vi "LOAD CELL FGV MAIN.vi"(7 "Enum":T2(ring), 8 "error in (no error)":errorcluster, 11 "main ref":T1) -> (0 "error IO":errorcluster)   [LabVIEW 2025]
uses:
  controls/LAB-IQ UI Data.ctl
  lib/hps_ft.dll
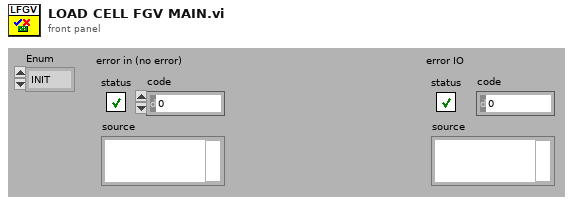
[diagram p1: front panel]
types:
  T1 = typedef "LAB-IQ UI Data.ctl" = cluster{"Main Home Screen":cluster{"GUI":refnum<vi>, "Platform Settings":refnum<vi>, "Configure":refnum<vi>, "Home":refnum<vi>, "EXIT":refnum<vi>, "service 2":refnum<vi>, "MainPage":refnum<vi>, "Analysis":refnum<vi>}, "Platform Settings":cluster{"mm/s  Surge":refnum<vi>, "Update Surge Speed":refnum<vi>, "Drive Error":refnum<vi>, "Disable Axis Jog Soft Limits":refnum<vi>, "mm/s  Sway":refnum<vi>, "Sway and Surge COM Status":refnum<vi>, "Heave COM Status":refnum<vi>, "Enable Platform":refnum<vi>, "Surge Forward Main":refnum<vi>, "Sway Right Main":refnum<vi>, "Sway Left Main":refnum<vi>, "Heave Down Main":refnum<vi>, "Heave Up main":refnum<vi>, "Update Sway Speed":refnum<vi>, "Update Heave Speed":refnum<vi>, "mm/s Heave":refnum<vi>, "mm/sec":refnum<vi>, "mm":refnum<vi>, "Surge Backward Main":refnum<vi>}, "Analysis Screen":cluster{"Analysis Home":refnum<vi>, "Surface Analysis":refnum<vi>, "Imaging":refnum<vi>, "Image Analysis":refnum<vi>, "Post Analysis":refnum<vi>}, "Config Screen":cluster{"Select Load Head":refnum<vi>, "Notes :":refnum<vi>, "FILE":refnum<vi>, "Sample ID :":refnum<vi>, "Operator ID :":refnum<vi>, "Operator Name :":refnum<vi>, "Auto":refnum<vi>}, "Motion Module":cluster{"zNL":refnum<vi>, "NL disp":refnum<vi>, "Rotary Tab":refnum<vi>, "Motion Direction:  3":refnum<vi>, "E.Velocity 2":refnum<vi>, "e.v/ssr 2":refnum<vi>, "Enter Fixed E.Velocity 2":refnum<vi>, "Enter Final SRR 2":refnum<vi>, "Enter initial SRR 2":refnum<vi>, "Enter Fixed SRR 2":refnum<vi>, "Enter the Final E.Velocity (m/s) 2":refnum<vi>, "Enter initial E.Velocity (m/s) 2":refnum<vi>, "Final Speed (RPM) 3":refnum<vi>, "Initial Speed (RPM) 2":refnum<vi>, "Enter the Final Velocity (m/s) 3":refnum<vi>, "Enter initial Velocity (m/s)  3":refnum<vi>, "Ramp Up 2":refnum<vi>, "TEST SELECTION":refnum<vi>, "SPEED SELECTION : ":refnum<vi>, "Angular Oscillation Set":refnum<vi>, "Traction":refnum<vi>, "Step Speed":refnum<vi>, "StepTable For Load-Speed":refnum<vi>, "StepTable For Speed":refnum<vi>, "Surge Forward MM":refnum<vi>, "Surge Backward MM":refnum<vi>, "M3 Image":refnum<vi>, "String 39":refnum<vi>, "Sway Left MM":refnum<vi>, "Sway Right MM":refnum<vi>, "Disable Axis Jog Soft Limits":refnum<vi>, "mm":refnum<vi>, "Heave Down MM":refnum<vi>, "Heave Up MM":refnum<vi>, "Wear Track Diameter (mm)":refnum<vi>, "Set WTD":refnum<vi>, "HomeScratch":refnum<vi>, "HomeRot":refnum<vi>, "PlaceModule":refnum<vi>, "Enter the Angle (Deg)":refnum<vi>, "Enter the Frequency (Hz)":refnum<vi>, "Motion Mode:":refnum<vi>, "LR Sway":refnum<vi>, "Rot Hor":refnum<vi>, "Scratch":refnum<vi>, "LR Cam":refnum<vi>, "MMBack":refnum<vi>, "MMNext":refnum<vi>, "Rot Ver":refnum<vi>, "Rotary Module Selection":refnum<vi>, "calculate rotary":refnum<vi>, "SPEED SELECTION : rotary":refnum<vi>, "Import 2":refnum<vi>, "Save 2":refnum<vi>, "File Path :  2":refnum<vi>, "String 45":refnum<vi>, "StepTable For Speed 3":refnum<vi>, "Enter the Speed(mm/sec)":refnum<vi>, "Enter the Speed(RPM)":refnum<vi>, "Enter Scratch Speed (mm/s):":refnum<vi>, "SwaySpeed Set":refnum<vi>, "Scartch Offset":refnum<vi>, "Motion type:":refnum<vi>, "HomeScratch 2":refnum<vi>, "Enter Scratch length (mm):":refnum<vi>, "Wear Track Diameter":refnum<vi>, "Rotary Speed Exced":refnum<vi>, "Scratch Mode":refnum<vi>, "No of Scratch":refnum<vi>}, "Environmental control":cluster{"Humidity  Status  3":refnum<vi>, "Low Temp  Status  2":refnum<vi>, "TK4 status 2":refnum<vi>, "Stage Temperature":refnum<vi>, "Sample Temperature":refnum<vi>, "Humidity (Amb)":refnum<vi>, "Clear List":refnum<vi>, "Add to list":refnum<vi>, "Wear":refnum<vi>, "Vibration":refnum<vi>, "Humidity (Chamber)":refnum<vi>, "Temperature (Chamber)":refnum<vi>, "ECR ":refnum<vi>, "Temperature (Amb)":refnum<vi>, "Microphone":refnum<vi>, "Acoustic Emission 3":refnum<vi>, "SNext":refnum<vi>, "APBack":refnum<vi>, "Enter the Temperature (°C):":refnum<vi>, "Enter the Stage \nTemperature (°C):":refnum<vi>, "Enter the Humidity (%Rh):":refnum<vi>, "Low Temp":refnum<vi>, "High Temp":refnum<vi>, "Humidity":refnum<vi>, "Sensors Picked":refnum<vi>}, "About Screen":cluster{"Password":refnum<vi>, "Home Service":refnum<vi>, "Advanced Setting":refnum<vi>, "About Tab":refnum<vi>, "ECR Port:":refnum<vi>, "Ramp Port:":refnum<vi>, "Installation/Replacement completed":refnum<vi>, "Loahead":refnum<vi>, "Heave and Surge COM Port:":refnum<vi>, "Sway COM Port:":refnum<vi>, "Temp Modbus:":refnum<vi>, "Humidity Port:":refnum<vi>, "Edit Gain Constants":refnum<vi>, "Save Gain Constants":refnum<vi>}, "Main Screen":cluster{"Main Screen Tab":refnum<vi>, "Angle and Frequency":refnum<vi>, "Stroke (mm)":refnum<vi>, "Angle (Deg)":refnum<vi>, "Main Speed Tab":refnum<vi>, "MTM MOTOR DISPLAY":refnum<vi>, "Disc Speed (m/sec)":refnum<vi>, "Ball Speed (m/sec)":refnum<vi>, "Disc Speed (RPM)":refnum<vi>, "Ball Speed (RPM)":refnum<vi>, "SPEED TAB":refnum<vi>, "Speed (m/sec)":refnum<vi>, "Set Speed (m/sec)":refnum<vi>, "Speed (RPM)":refnum<vi>, "Set Speed":refnum<vi>, "Time Tab":refnum<vi>, "Time ( HH:MM:SS ) 2":refnum<vi>, "Test Duration":refnum<vi>, "Test Duration 4":refnum<vi>, "TEST CYCLE":refnum<vi>, "TOTAL CYCLES":refnum<vi>, "Set Load (N)":refnum<vi>, "Temp Tabs":refnum<vi>, "Heater":refnum<vi>, "TK4 status":refnum<vi>, "ChamberTemp":refnum<vi>, "SetTmp":refnum<vi>, "Controller  Status":refnum<vi>, "ChamberTemp 2":refnum<vi>, "SetTmp 2":refnum<vi>, "Controller  Status 2":refnum<vi>, "ChamberTemp 3":refnum<vi>, "SetTmp 3":refnum<vi>, "Cooling":refnum<vi>, "Load Communication":refnum<vi>, "Ambient \nTemperature":refnum<vi>, "HumCOMStatus":refnum<vi>, "Ambient\n Humidity":refnum<vi>, "Freq (Hz)":refnum<vi>, "Load En":refnum<vi>, "NLt":refnum<vi>, "zNL 2":refnum<vi>, "Humidity On":refnum<vi>, "humidity disp":refnum<vi>, "Set Humidity":refnum<vi>, "NL disp 2":refnum<vi>, "Humidity On 2":refnum<vi>, "humidity disp 2":refnum<vi>, "Set Humidity 2":refnum<vi>, "NL disp 3":refnum<vi>, "AppLoadSeq scratch":refnum<vi>, "Stop Scratch":refnum<vi>, "ClrLog":refnum<vi>, "Trip Log":refnum<vi>, "STOP":refnum<vi>, "Start Test":refnum<vi>, "Test status":refnum<vi>, "AR Led":refnum<vi>, "Data":refnum<vi>, "Health":refnum<vi>, "Sway COM Status":refnum<vi>, "Heave COM Status":refnum<vi>, "Grp Tab":refnum<vi>, "Sub Graph":refnum<vi>, "SD (mm)":refnum<vi>, "Siliding distance Reset Graph":refnum<vi>, "SDGp":refnum<vi>, "Humidity Reset Graph":refnum<vi>, "HumrGp":refnum<vi>, "Acoustic Emission (mV)":refnum<vi>, "Aqucostic Reset Graph":refnum<vi>, "gACQUOS":refnum<vi>, "ECR RESET":refnum<vi>, "ECR":refnum<vi>, "Temperature Reset":refnum<vi>, "Acoustic Emission (mV) 2":refnum<vi>, "Aqucostic Reset Graph 2":refnum<vi>, "gACQUOS 2":refnum<vi>, "ECR RESET 2":refnum<vi>, "ECR 2":refnum<vi>, "Temperature Reset 2":refnum<vi>, "Temperature (deg c)":refnum<vi>, "Speed Reset Graph":refnum<vi>, "Speed Tab":refnum<vi>, "MTM DISC  SPEED":refnum<vi>, "MTM BALL SPEED":refnum<vi>, "speed mm/sec":refnum<vi>, "Hymidity":refnum<vi>, "Humidity Disable trip":refnum<vi>, "CoF Trip  2":refnum<vi>, "Depth Trip":refnum<vi>, "Weart Deapth":refnum<vi>, "Depth Reset Graph":refnum<vi>, "Weart":refnum<vi>, "Depthz":refnum<vi>, "Depth (µm)":refnum<vi>, "WearGp":refnum<vi>, "NL Trip 2":refnum<vi>, "Load pid":refnum<vi>, "Load Disable Trip":refnum<vi>, "Load Reset Graph":refnum<vi>, "NL Display 4":refnum<vi>, "Main Chart 3":refnum<vi>, "BACK":refnum<vi>, "Depth Trip 2":refnum<vi>, "COF TRIP ":refnum<vi>, "Friction Force (N)":refnum<vi>, "FF Reset Graph":refnum<vi>, "FF Disable Trip":refnum<vi>, "FF TRIP":refnum<vi>, "COF Disable Trip":refnum<vi>, "COF Reset Graph":refnum<vi>, "Start Test Temp":refnum<vi>, "zFF":refnum<vi>, "Friction Force (N) Graph":refnum<vi>, "Coefficient of Friction":refnum<vi>, "Scratch Start Test":refnum<vi>, "FF Tab":refnum<vi>, "Cyclic Friction Force (N)":refnum<vi>, "CZ FF":refnum<vi>, "Cyclic Friction Force (N) Graph":refnum<vi>, "Cyclic Coefficient of Friction":refnum<vi>, "Cyclic FF TRIP":refnum<vi>, "Cyclic FF Disable Trip":refnum<vi>, "cyclic COF Disable Trip":refnum<vi>, "cyclic COF TRIP":refnum<vi>, "cyclic COF Reset Graph":refnum<vi>, "Cyclic FF Reset Graph":refnum<vi>, "Test Trip":refnum<vi>, "Multi Scratch Pass":refnum<vi>}, "Loading":cluster{"Indentation":refnum<vi>, "Reference Sample":refnum<vi>, "Load Cell Communication Slide":refnum<vi>, "com 3":refnum<vi>, "com":refnum<vi>, "DecaForce COM Status":refnum<vi>, "Update":refnum<vi>, "Clear 3":refnum<vi>, "seq":refnum<vi>, "Stribeck table":refnum<vi>, "Stribeck Table  For loading":refnum<vi>, "Loading Mode":refnum<vi>, "Enter the Final Load (N)":refnum<vi>, "Enter the CoF Trip":refnum<vi>, "Enter the Friction Force Trip":refnum<vi>, "Enter the Normal load Trip":refnum<vi>, "Enter the Load  (N)":refnum<vi>, "KiloForce":refnum<vi>, "DecaForce ":refnum<vi>, "MicroForce":refnum<vi>, "LHBack":refnum<vi>, "LHNext":refnum<vi>, "Enter the Loading Rate (N/min)":refnum<vi>, "Message":refnum<vi>, "Warning 2":refnum<vi>, "SSP 0.75":refnum<vi>, "SSP 0.5":refnum<vi>, "SSP 0.3":refnum<vi>, "Warning":refnum<vi>, "gui GIF":refnum<vi>, "Communication is established":refnum<vi>, "AppLoad 4":refnum<vi>, "Multipoint":refnum<vi>, "Load Selection":refnum<vi>}, "PID":cluster{"Ramp MulFac":refnum<vi>, "pulses LoadDiffRamp(2..10)":refnum<vi>, "PulseControlRamp(diff<=3N)":refnum<vi>, "SetLoadDeadband(%) Load(0-10N)":refnum<vi>, "PID gains out delay (microForce)":refnum<vi>, "Ramp":refnum<vi>, "Gain 2":refnum<vi>, "pulses LoadDiff(2..10)":refnum<vi>, "pulses LoadDiff(11..50)":refnum<vi>, "PulseControl(diff<=3N)":refnum<vi>, "SetLoadDeadband(%)  2":refnum<vi>, "Dummy Run":refnum<vi>, "Vertical load (N)":refnum<vi>, "AutoTune":refnum<vi>, "Offset 3 ":refnum<vi>, "apply load":refnum<vi>, "Offset  3":refnum<vi>, "apply load 2":refnum<vi>, "Enter ByPass Load":refnum<vi>, "reinit 3":refnum<vi>, "output range delay":refnum<vi>, "PID gains out delay":refnum<vi>, "Bypass Load":refnum<vi>, "pulsesSent":refnum<vi>, "pulses ":refnum<vi>, "actpid":refnum<vi>, "gFF Rot":refnum<vi>, "pulses LoadDiff(21..1000)":refnum<vi>, "Delay":refnum<vi>, "deadband":refnum<vi>}, "Config Parameters":cluster{"Tab Control 3":refnum<vi>, "Tab Control 19":refnum<vi>, "SAMPLES":refnum<vi>, "Re-initilaize":refnum<vi>, "Filter ON/OFF":refnum<vi>, "TracHomeSurgeOffsetCounts 10MM":refnum<vi>, "TracHomeSwayOffsetCounts 10MM":refnum<vi>, "Acoustic Emission:":refnum<vi>, "Apply Filter (FF)":refnum<vi>, "Filter% 2":refnum<vi>, "Apply Filter (Load)":refnum<vi>, "Filter% ":refnum<vi>, "Sway distance (mm)":refnum<vi>, "Surge distance (mm)":refnum<vi>, "DataSavingLoopDelay(ms)":refnum<vi>, "SAVE 2":refnum<vi>, "Enter Distance":refnum<vi>, "Sway Counts:":refnum<vi>, "Distance (mm): 3":refnum<vi>, "Surge Counts:":refnum<vi>, "Distance (mm): 2":refnum<vi>, "Distance (mm):":refnum<vi>, "Heave Counts:":refnum<vi>, "LRMHomeSurgeOffsetCounts":refnum<vi>, "LRMHomeSwayOffsetCounts":refnum<vi>, "TracHomeSurgeOffsetCounts 20MM":refnum<vi>, "TracHomeSwayOffsetCounts 20MM":refnum<vi>, "RotHomeSwayOffsetCounts":refnum<vi>, "RotHomeSurgeOffsetCounts":refnum<vi>, "Heave distance":refnum<vi>, "Zmm":refnum<vi>, "Heave Pulses/mm":refnum<vi>, "Surge Pulses/mm":refnum<vi>, "Sway Pulses/mm":refnum<vi>, "Heave Pitch":refnum<vi>, "Surge Pitch":refnum<vi>, "Sway Pitch":refnum<vi>, "Heave PPR":refnum<vi>, "Surge PPR":refnum<vi>, "Sway PPR":refnum<vi>, "Tab Control 5":refnum<vi>, "Tab Control 14":refnum<vi>, "Tab Control 26":refnum<vi>, "AE":refnum<vi>, "Heave Loop Delay":refnum<vi>, "Heave PID Speed":refnum<vi>, "Surge Jog Speed":refnum<vi>, "Heave Jog Speed":refnum<vi>, "Sway Loop Delay":refnum<vi>, "Sway PID Speed":refnum<vi>, "Sway Jog Speed":refnum<vi>}, "Loading Com Port":cluster{"ClearAll":refnum<vi>, "Mz(Nm)":refnum<vi>, "My(Nm)":refnum<vi>, "Mx(Nm)":refnum<vi>, "Save Dwell":refnum<vi>, "Mx ":refnum<vi>, "My ":refnum<vi>, "Mz":refnum<vi>, "Fx(N)":refnum<vi>, "Fy(N)":refnum<vi>, "Fz(N)":refnum<vi>, "ZeroAll":refnum<vi>, "Acq Delay (ms)":refnum<vi>, "Burst Delay (ms)":refnum<vi>, "model":refnum<vi>, "SN":refnum<vi>, "FFx(N)":refnum<vi>, "Sensor IP":refnum<vi>, "Port":refnum<vi>, "FFy(N)":refnum<vi>, "Load(N)":refnum<vi>, "delete Handle":refnum<vi>, "Create Handle":refnum<vi>, "ft_data":refnum<vi>, "ft_range":refnum<vi>, "ft_data 2":refnum<vi>, "stop 6":refnum<vi>, "running_flag":refnum<vi>, "ft_udp_handle":refnum<vi>, "get-data-return":refnum<vi>, "get-range-return":refnum<vi>, "zero-return":refnum<vi>, "filter-return":refnum<vi>, "initial-return":refnum<vi>, "deleteHandle-result":refnum<vi>, "Load Cell Temp":refnum<vi>}, "Heave AND Surge":cluster{"SURGE POSE":refnum<vi>, "error out Read":refnum<vi>, "HEAVE POSE":refnum<vi>, "State":refnum<vi>, "Homed":refnum<vi>, "Sequence ID":refnum<vi>, "error out Write":refnum<vi>, "faultCode":refnum<vi>, "Ack ID":refnum<vi>, "SPEED":refnum<vi>, "Distance":refnum<vi>, "Mode Command":refnum<vi>, "Heave and Surge Read":refnum<vi>, "Read Heave Temp":refnum<vi>, "Spare 15":refnum<vi>, "Spare 14":refnum<vi>, "Spare 13":refnum<vi>, "Spare 12":refnum<vi>, "Spare 11":refnum<vi>, "Spare 10":refnum<vi>, "Spare 9":refnum<vi>, "Spare 8":refnum<vi>, "Spare 7":refnum<vi>, "Spare 6":refnum<vi>, "Spare 5":refnum<vi>, "Spare 4":refnum<vi>, "Spare 2":refnum<vi>, "Spare 1":refnum<vi>, "Node Id":refnum<vi>, "Spare 3":refnum<vi>, "SPARE 4":refnum<vi>, "SPARE 3":refnum<vi>, "SPARE 2":refnum<vi>, "SPARE 1":refnum<vi>, "fwMajor":refnum<vi>, "fwMinor":refnum<vi>, "Manual Write":refnum<vi>, "Heave and Surge Write":refnum<vi>}, "New PID LOGIC":cluster{"Fine Tune Zone":refnum<vi>, "PID SDelay":refnum<vi>, "Max_pos_limit":refnum<vi>, "Min_pos_limit":refnum<vi>, "i_limit":refnum<vi>, "pct_scale":refnum<vi>, "Deadband":refnum<vi>, "Kd":refnum<vi>, "Ki":refnum<vi>, "Kp":refnum<vi>, "Current Position":refnum<vi>, "Set Load":refnum<vi>, "Current Load":refnum<vi>, "Pulse delta":refnum<vi>, "Init Step":refnum<vi>, "Max Step Linit":refnum<vi>}, "SWAY ":cluster{"fwMajor":refnum<vi>, "Homed":refnum<vi>, "Rotary POSE":refnum<vi>, "State":refnum<vi>, "SWAY POSE":refnum<vi>, "Ack ID":refnum<vi>, "faultCode":refnum<vi>, "Node Id":refnum<vi>, "fwMinor":refnum<vi>, "Spare 6":refnum<vi>, "Spare 5":refnum<vi>, "Spare 4":refnum<vi>, "Spare 3":refnum<vi>, "Spare 2":refnum<vi>, "Spare 1":refnum<vi>, "Spare 7":refnum<vi>, "SPARE  5":refnum<vi>, "error out Write  SWAY ":refnum<vi>, "error out Read SWAY ":refnum<vi>, "Manual Write SWAY ":refnum<vi>, "SWAY WRITE":refnum<vi>, "SPARE  4":refnum<vi>, "SPARE  3":refnum<vi>, "SPARE 2":refnum<vi>, "SPARE 1":refnum<vi>, "Spare 15":refnum<vi>, "Spare 14":refnum<vi>, "Spare 13":refnum<vi>, "Spare 12":refnum<vi>, "Spare 11":refnum<vi>, "Spare 9":refnum<vi>, "Spare 8":refnum<vi>, "SPEED":refnum<vi>, "Distance":refnum<vi>, "Mode Command":refnum<vi>, "Sequence ID":refnum<vi>, "SWAY READ":refnum<vi>, "Spare 10":refnum<vi>, "Read SWAY Temp":refnum<vi>}, "Analysis Screen":cluster{"Analysis Home":refnum<vi>, "Refresh 2":refnum<vi>, "MEAN 4":refnum<vi>, "SD 4":refnum<vi>, "VARIANCE 4":refnum<vi>, "MEAN  3":refnum<vi>, "SD  3":refnum<vi>, "VARIANCE  3":refnum<vi>, "MEAN 2":refnum<vi>, "SD  2":refnum<vi>, "VARIANCE 2":refnum<vi>, "MEAN":refnum<vi>, "SD":refnum<vi>, "VARIANCE":refnum<vi>, "File 4 Discription":refnum<vi>, "OPEN 4":refnum<vi>, "File Name 4":refnum<vi>, "OPEN 3":refnum<vi>, "File 3 Discription":refnum<vi>, "File Name 3":refnum<vi>, "Y-AXIS":refnum<vi>, "X-AXIS":refnum<vi>, "XY Graph":refnum<vi>, "File Name 2":refnum<vi>, "File Name 1":refnum<vi>, "OPEN 2":refnum<vi>, "OPEN 1":refnum<vi>, "File 1 Discription ":refnum<vi>, "File 2 Discription":refnum<vi>}}
  T2 = enum16{"INIT", "SETLOWPASSFILTER", "SETZERO", "GETSENSORINFO", "GETRANGE", "ZEROALL", "READDATA", "UNINITIAL", "DELETEHANDLE"}
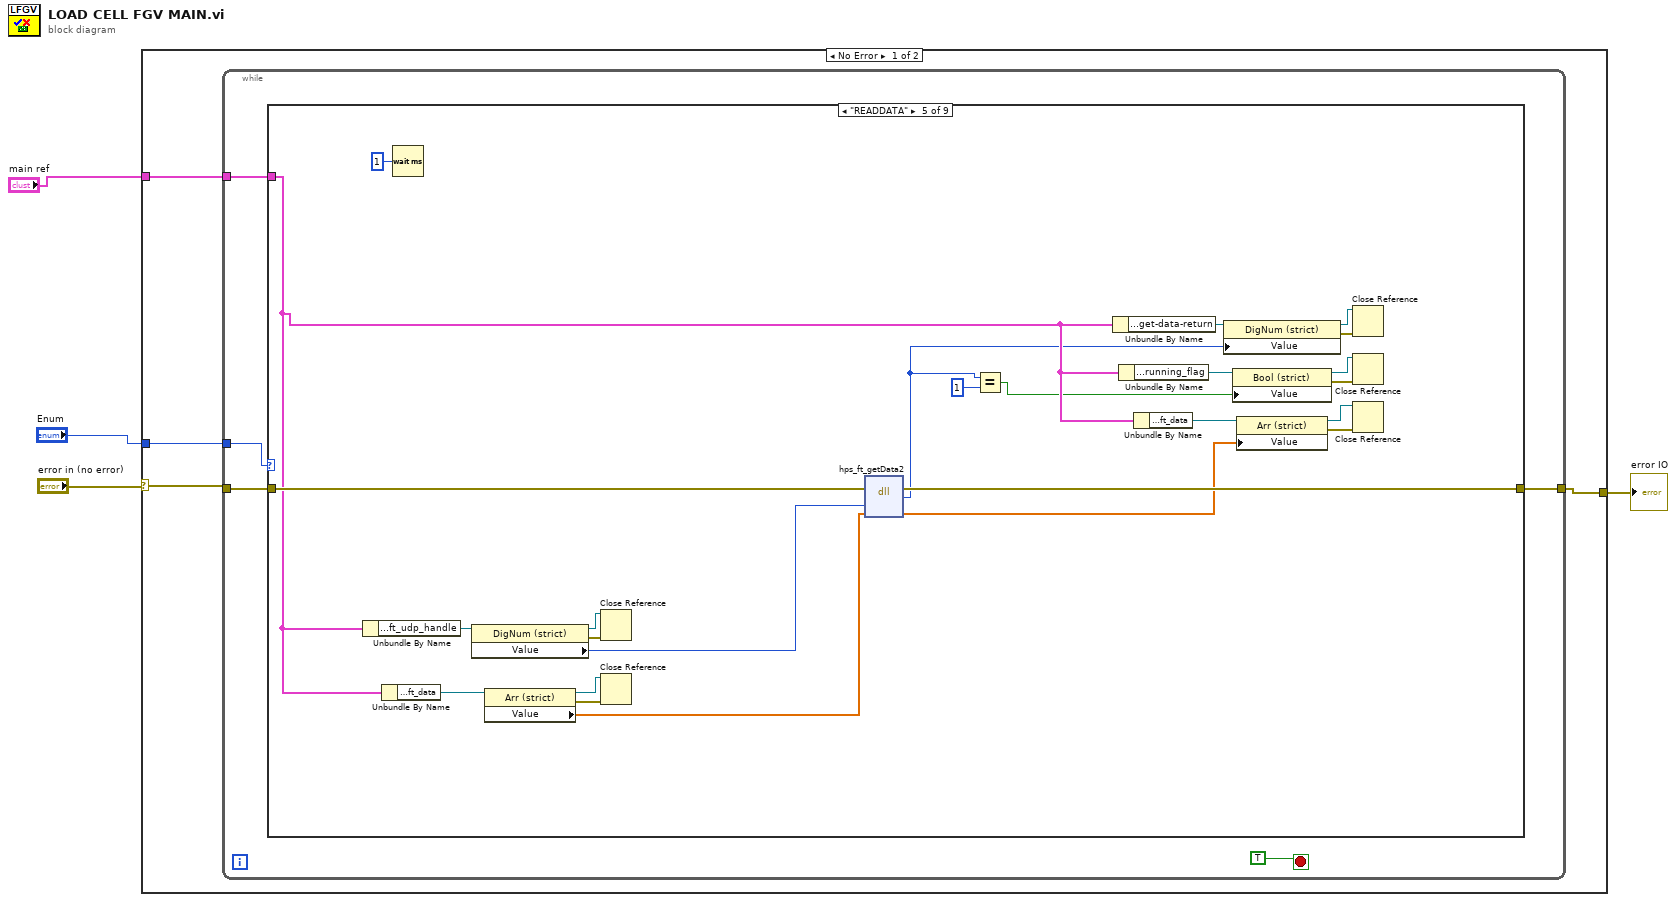
[diagram p0: block diagram]
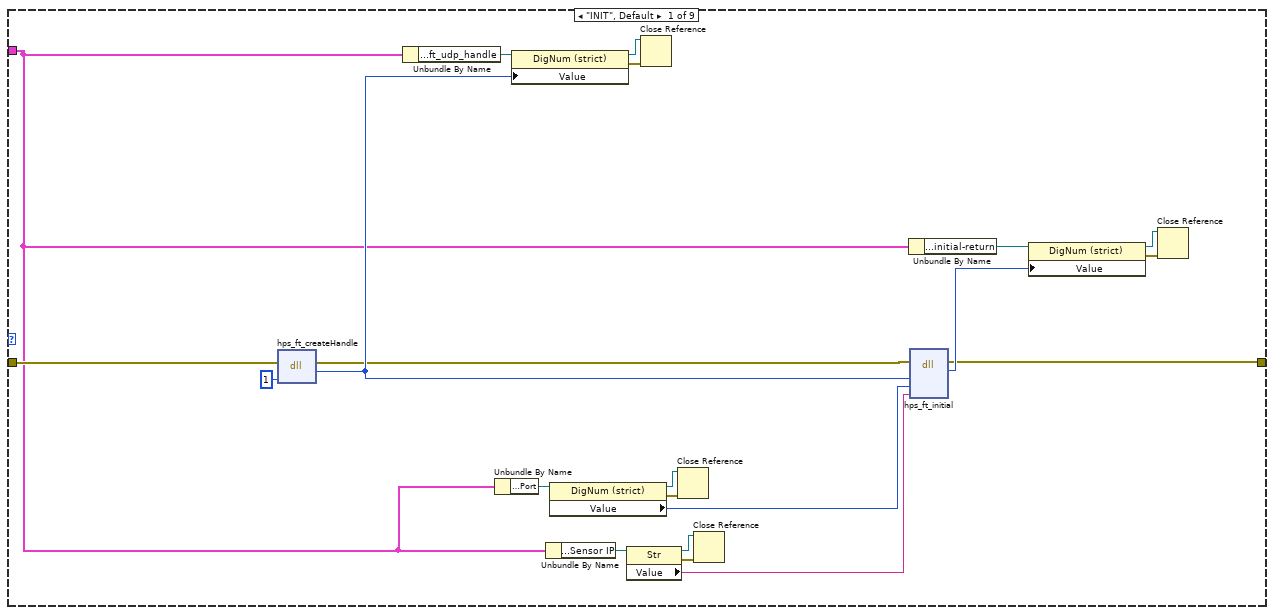
[diagram p2: hidden frame]
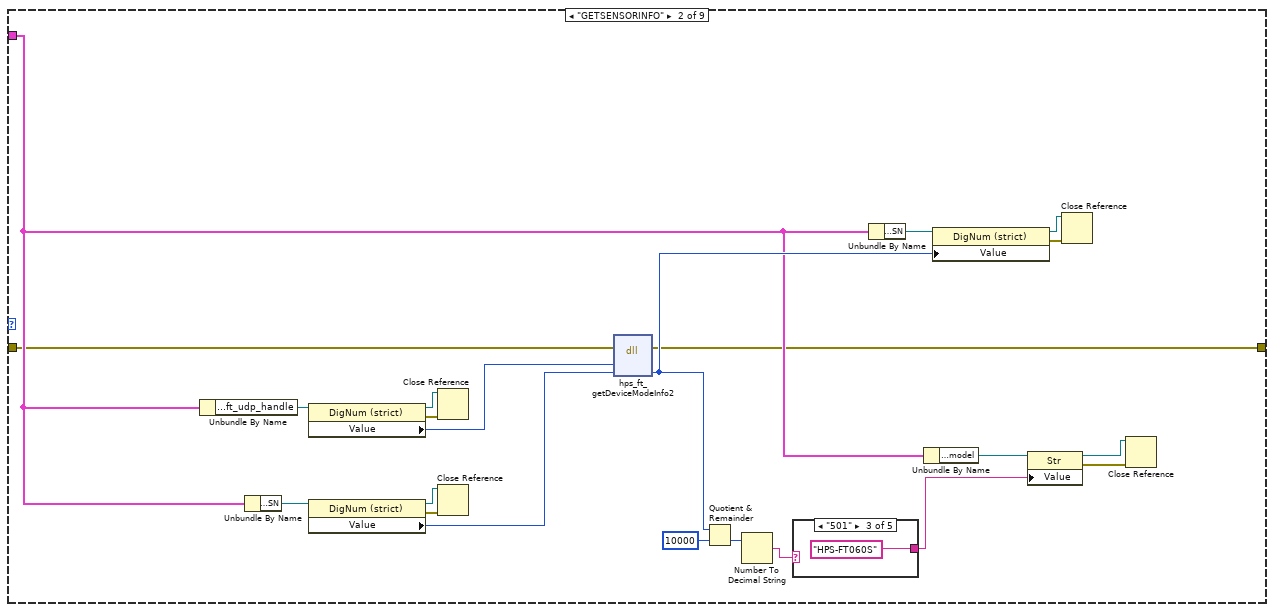
[diagram p3: hidden frame]
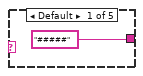
[diagram p4: hidden frame]
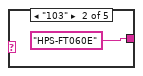
[diagram p5: hidden frame]
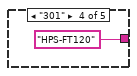
[diagram p6: hidden frame]
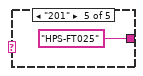
[diagram p7: hidden frame]
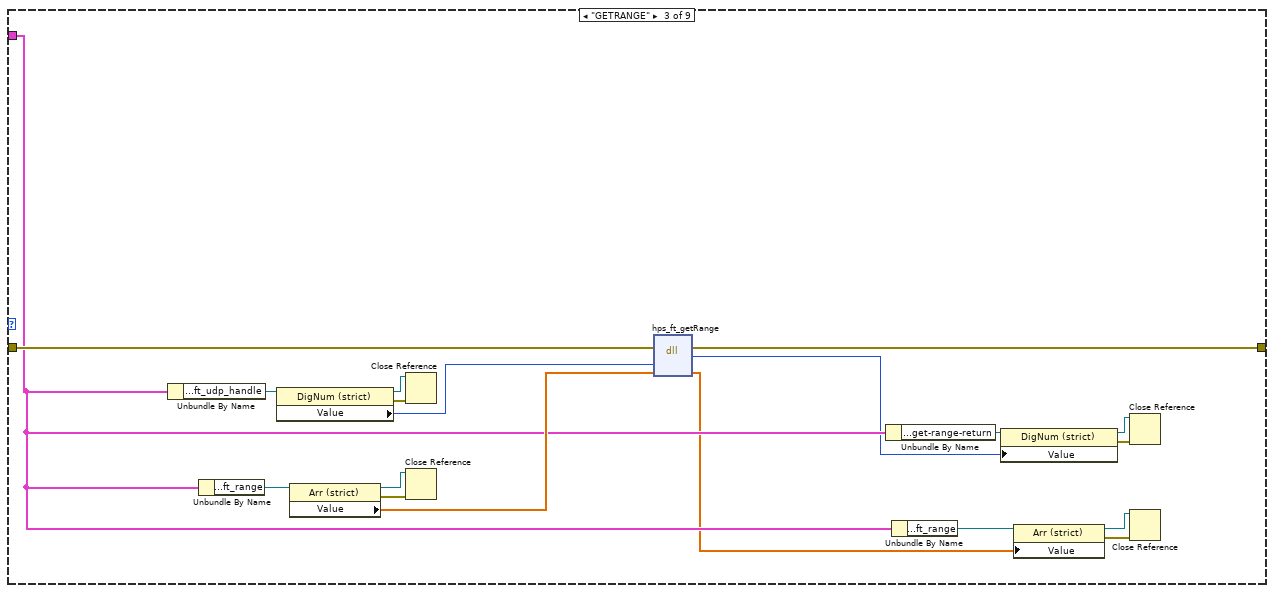
[diagram p8: hidden frame]
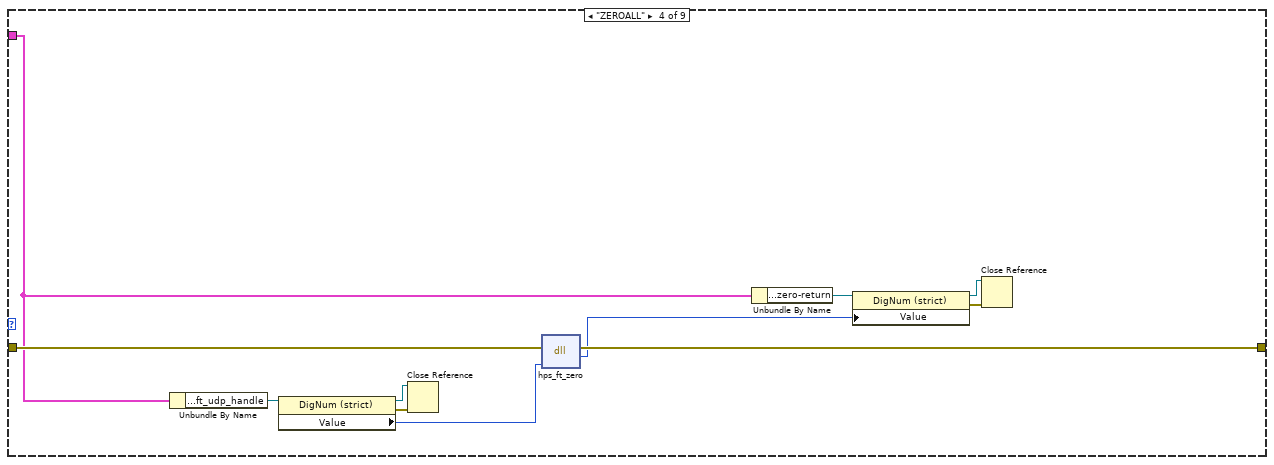
[diagram p9: hidden frame]
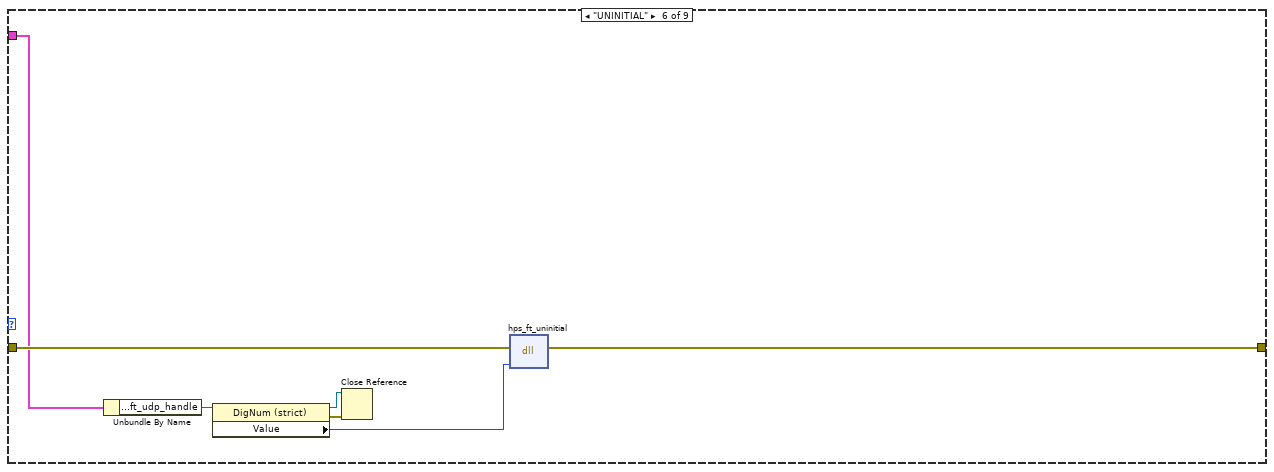
[diagram p10: hidden frame]
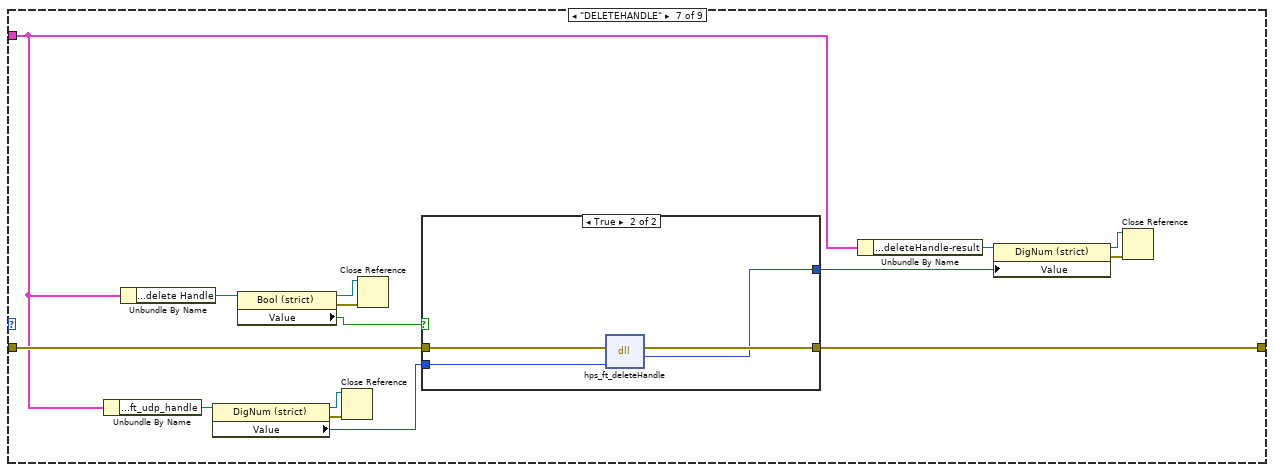
[diagram p11: hidden frame]
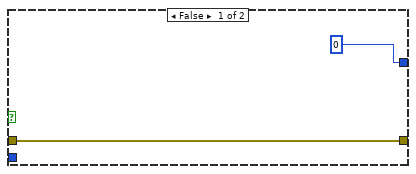
[diagram p12: hidden frame]
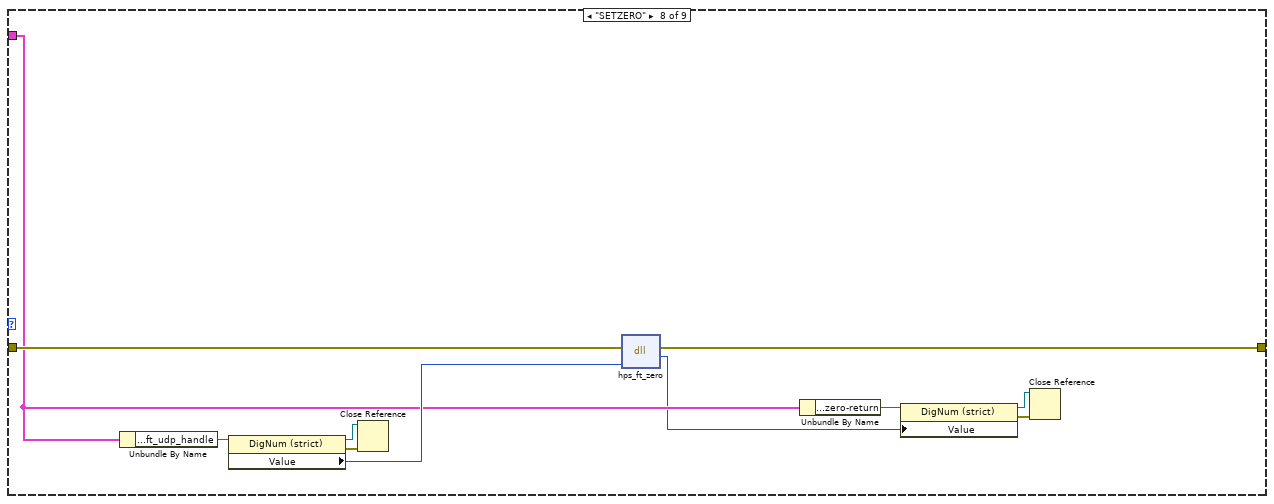
[diagram p13: hidden frame]
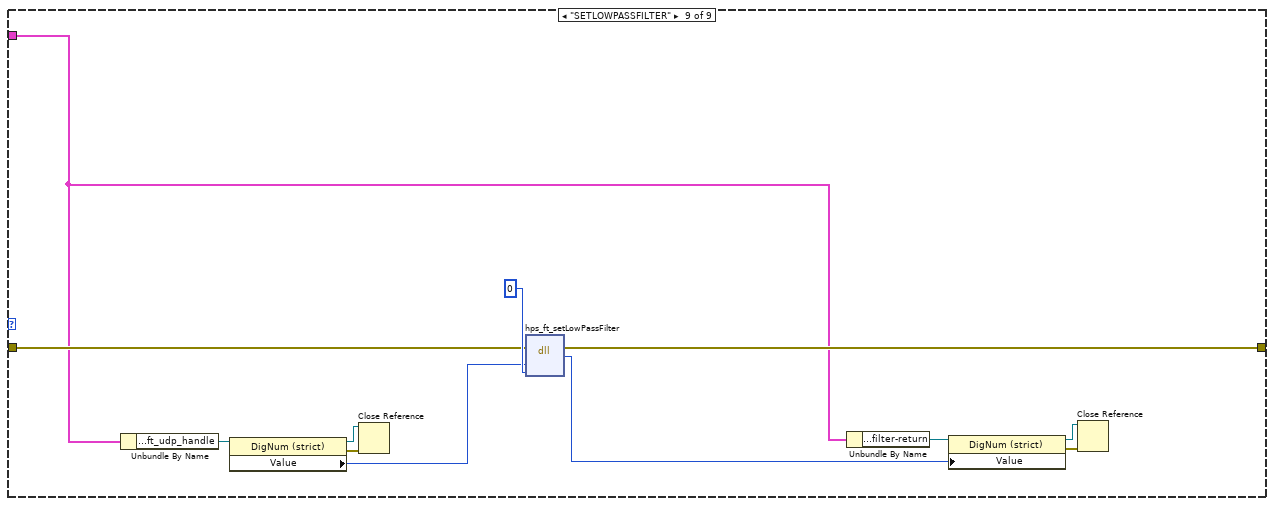
[diagram p14: hidden frame]
diagram:
  n1 = case shown="No Error" "error in (no error)" {
    selector: "error in (no error)" -> [w8 _]
    tunnel: [w7 _] -> w3
    tunnel: "Enum" -> [w6 _]
    tunnel: "main ref" -> [w5 _]
    frame No Error {
      n2 = while {
        tunnel: [w11] -> w7
        tunnel: w8 -> [w12]
        tunnel: w6 -> [w10]
        tunnel: w5 -> [w9]
        stop <- TRUE ("stop") stop-if-true
        n3 = case shown="\"READDATA\"" w10 {
          tunnel: w12 -> [w21 w36 w80 w91 w114 w123 w138 w155 w166]
          tunnel: [w14 w35 w79 w90 w113 w122 w137 w145 w165] -> w11
          tunnel: w9 -> [w16 w38 w64 w82 w96 w117 w125 w147 w157]
          frame "INIT", Default {
            n4 = dll-call lib="D:/LAB-IQ 150/lib/hps_ft.dll" fn="hps_ft_createHandle"(error in=w21, "1(UDP)"=1) -> (error out=w20:errorcluster, "return type"=w30:i32)  [unwired: 3 in, 1 out]
            n5 = Unbundle By Name(w16) -> ("Loading Com Port.ft_udp_handle"=w31:refnum<vi>)
            n6 = Unbundle By Name(w16) -> ("Loading Com Port.Port"=w25:refnum<vi>)
            n7 = property class="DigNum (strict)"(reference=w31, "Value"=w30) -> (reference out=w33:refnum<vi>, error out=w32:errorcluster)  [unwired: 1 in]
            n8 = Unbundle By Name(w16) -> ("Loading Com Port.Sensor IP"=w29:refnum<vi>)
            n9 = property class="DigNum (strict)"(reference=w25) -> (reference out=w24:refnum<vi>, error out=w26:errorcluster, "Value"=w23:i32)  [unwired: 1 in]
            n10 = property class="Str"(reference=w29) -> (reference out=w27:refnum<vi>, error out=w28:errorcluster, "Value"=w22:string)  [unwired: 1 in]
            n11 = Close Reference(reference=w33, error in (no error)=w32) -> ()  [unwired: 1 out]
            n12 = Close Reference(reference=w24, error in (no error)=w26) -> ()  [unwired: 1 out]
            n13 = Close Reference(reference=w27, error in (no error)=w28) -> ()  [unwired: 1 out]
            n14 = Unbundle By Name(w16) -> ("Loading Com Port.initial-return"=w19:refnum<vi>)
            n15 = dll-call lib="D:/LAB-IQ 150/lib/hps_ft.dll" fn="hps_ft_initial"(error in=w20, "handle"=w30, "port"=w23, "IP"=w22) -> (error out=w14:errorcluster, "return type"=w15:i32)  [unwired: 5 in, 1 out]
            n16 = property class="DigNum (strict)"(reference=w19, "Value"=w15) -> (reference out=w17:refnum<vi>, error out=w18:errorcluster)  [unwired: 1 in]
            n17 = Close Reference(reference=w17, error in (no error)=w18) -> ()  [unwired: 1 out]
          }
          frame "GETSENSORINFO" {
            n18 = Unbundle By Name(w38) -> ("Loading Com Port.ft_udp_handle"=w51:refnum<vi>)
            n19 = Unbundle By Name(w38) -> ("Loading Com Port.SN"=w48:refnum<vi>)
            n20 = property class="DigNum (strict)"(reference=w51) -> (reference out=w53:refnum<vi>, error out=w52:errorcluster, "Value"=w47:i32)  [unwired: 1 in]
            n21 = property class="DigNum (strict)"(reference=w48) -> (reference out=w50:refnum<vi>, error out=w49:errorcluster, "Value"=w46:i32)  [unwired: 1 in]
            n22 = Close Reference(reference=w53, error in (no error)=w52) -> ()  [unwired: 1 out]
            n23 = Close Reference(reference=w50, error in (no error)=w49) -> ()  [unwired: 1 out]
            n24 = dll-call lib="D:/LAB-IQ 150/lib/hps_ft.dll" fn="hps_ft_getDeviceModeInfo2"(error in=w36, "handle"=w47, "sensor_info"=w46) -> (error out=w35:errorcluster, "sensor_info"=w42:i32)  [unwired: 4 in, 1 out]
            n25 = Quotient & Remainder(x=w42, y=10000) -> (floor(x/y)=w56:i32)  [unwired: 1 out]
            n26 = Number To Decimal String(number=w56) -> (decimal integer string=w54:string)  [unwired: 1 in]
            n27 = case shown="\"501\"" w54 {
              tunnel: ["#####" "HPS-FT060E" "HPS-FT060S" "HPS-FT120" "HPS-FT025"] -> w37
              frame Default {
              }
              frame "103" {
              }
              frame "501" {
              }
              frame "301" {
              }
              frame "201" {
              }
            }
            n28 = Unbundle By Name(w38) -> ("Loading Com Port.SN"=w45:refnum<vi>)
            n29 = Unbundle By Name(w38) -> ("Loading Com Port.model"=w39:refnum<vi>)
            n30 = property class="DigNum (strict)"(reference=w45, "Value"=w42) -> (reference out=w43:refnum<vi>, error out=w44:errorcluster)  [unwired: 1 in]
            n31 = property class="Str"(reference=w39, "Value"=w37) -> (reference out=w41:refnum<vi>, error out=w40:errorcluster)  [unwired: 1 in]
            n32 = Close Reference(reference=w43, error in (no error)=w44) -> ()  [unwired: 1 out]
            n33 = Close Reference(reference=w41, error in (no error)=w40) -> ()  [unwired: 1 out]
          }
          frame "GETRANGE" {
            n34 = Unbundle By Name(w64) -> ("Loading Com Port.ft_udp_handle"=w76:refnum<vi>)
            n35 = Unbundle By Name(w64) -> ("Loading Com Port.ft_range"=w73:refnum<vi>)
            n36 = property class="DigNum (strict)"(reference=w76) -> (reference out=w78:refnum<vi>, error out=w77:errorcluster, "Value"=w72:i32)  [unwired: 1 in]
            n37 = property class="Arr (strict)"(reference=w73) -> (reference out=w75:refnum<vi>, error out=w74:errorcluster, "Value"=w71:dbl[])  [unwired: 1 in]
            n38 = Close Reference(reference=w78, error in (no error)=w77) -> ()  [unwired: 1 out]
            n39 = Close Reference(reference=w75, error in (no error)=w74) -> ()  [unwired: 1 out]
            n40 = dll-call lib="D:/LAB-IQ 150/lib/hps_ft.dll" fn="hps_ft_getRange"(error in=w80, "handle"=w72, "fi_data"=w71) -> (error out=w79:errorcluster, "return type"=w62:i32, "fi_data"=w63:dbl[])  [unwired: 3 in, 1 out]
            n41 = Unbundle By Name(w64) -> ("Loading Com Port.get-range-return"=w68:refnum<vi>)
            n42 = Unbundle By Name(w64) -> ("Loading Com Port.ft_range"=w65:refnum<vi>)
            n43 = property class="DigNum (strict)"(reference=w68, "Value"=w62) -> (reference out=w70:refnum<vi>, error out=w69:errorcluster)  [unwired: 1 in]
            n44 = property class="Arr (strict)"(reference=w65, "Value"=w63) -> (reference out=w67:refnum<vi>, error out=w66:errorcluster)  [unwired: 1 in]
            n45 = Close Reference(reference=w70, error in (no error)=w69) -> ()  [unwired: 1 out]
            n46 = Close Reference(reference=w67, error in (no error)=w66) -> ()  [unwired: 1 out]
          }
          frame "ZEROALL" {
            n47 = Unbundle By Name(w82) -> ("Loading Com Port.ft_udp_handle"=w87:refnum<vi>)
            n48 = property class="DigNum (strict)"(reference=w87) -> (reference out=w89:refnum<vi>, error out=w88:errorcluster, "Value"=w86:i32)  [unwired: 1 in]
            n49 = Close Reference(reference=w89, error in (no error)=w88) -> ()  [unwired: 1 out]
            n50 = dll-call lib="D:/LAB-IQ 150/lib/hps_ft.dll" fn="hps_ft_zero"(error in=w91, "handle"=w86) -> (error out=w90:errorcluster, "return type"=w81:i32)  [unwired: 3 in, 1 out]
            n51 = Unbundle By Name(w82) -> ("Loading Com Port.zero-return"=w83:refnum<vi>)
            n52 = property class="DigNum (strict)"(reference=w83, "Value"=w81) -> (reference out=w85:refnum<vi>, error out=w84:errorcluster)  [unwired: 1 in]
            n53 = Close Reference(reference=w85, error in (no error)=w84) -> ()  [unwired: 1 out]
          }
          frame "READDATA" {
            n54 = Unbundle By Name(w96) -> ("Loading Com Port.ft_udp_handle"=w110:refnum<vi>)
            n55 = Unbundle By Name(w96) -> ("Loading Com Port.ft_data"=w109:refnum<vi>)
            n56 = Wait (ms)(milliseconds to wait=u32 1) -> ()  [unwired: 1 out]
            n57 = property class="DigNum (strict)"(reference=w110) -> (reference out=w112:refnum<vi>, error out=w111:errorcluster, "Value"=w106:i32)  [unwired: 1 in]
            n58 = property class="Arr (strict)"(reference=w109) -> (reference out=w107:refnum<vi>, error out=w108:errorcluster, "Value"=w105:dbl[])  [unwired: 1 in]
            n59 = Close Reference(reference=w112, error in (no error)=w111) -> ()  [unwired: 1 out]
            n60 = Close Reference(reference=w107, error in (no error)=w108) -> ()  [unwired: 1 out]
            n61 = dll-call lib="D:/LAB-IQ 150/lib/hps_ft.dll" fn="hps_ft_getData2"(error in=w114, "handle"=w106, "fi_data"=w105) -> (error out=w113:errorcluster, "return type"=w95:i32, "fi_data"=w93:dbl[])  [unwired: 3 in, 1 out]
            n62 = Equal?(x=w95, y=1) -> (x = y?=w94:bool)
            n63 = Unbundle By Name(w96) -> ("Loading Com Port.get-data-return"=w104:refnum<vi>)
            n64 = Unbundle By Name(w96) -> ("Loading Com Port.running_flag"=w99:refnum<vi>)
            n65 = Unbundle By Name(w96) -> ("Loading Com Port.ft_data"=w98:refnum<vi>)
            n66 = property class="DigNum (strict)"(reference=w104, "Value"=w95) -> (reference out=w102:refnum<vi>, error out=w103:errorcluster)  [unwired: 1 in]
            n67 = property class="Bool (strict)"(reference=w99, "Value"=w94) -> (reference out=w101:refnum<vi>, error out=w100:errorcluster)  [unwired: 1 in]
            n68 = property class="Arr (strict)"(reference=w98, "Value"=w93) -> (reference out=w92:refnum<vi>, error out=w97:errorcluster)  [unwired: 1 in]
            n69 = Close Reference(reference=w102, error in (no error)=w103) -> ()  [unwired: 1 out]
            n70 = Close Reference(reference=w101, error in (no error)=w100) -> ()  [unwired: 1 out]
            n71 = Close Reference(reference=w92, error in (no error)=w97) -> ()  [unwired: 1 out]
          }
          frame "UNINITIAL" {
            n72 = Unbundle By Name(w117) -> ("Loading Com Port.ft_udp_handle"=w119:refnum<vi>)
            n73 = property class="DigNum (strict)"(reference=w119) -> (reference out=w121:refnum<vi>, error out=w120:errorcluster, "Value"=w118:i32)  [unwired: 1 in]
            n74 = Close Reference(reference=w121, error in (no error)=w120) -> ()  [unwired: 1 out]
            n75 = dll-call lib="D:/LAB-IQ 150/lib/hps_ft.dll" fn="hps_ft_uninitial"(error in=w123, "handle"=w118) -> (error out=w122:errorcluster)  [unwired: 4 in, 1 out]
          }
          frame "DELETEHANDLE" {
            n76 = Unbundle By Name(w125) -> ("Loading Com Port.ft_udp_handle"=w134:refnum<vi>)
            n77 = Unbundle By Name(w125) -> ("Loading Com Port.delete Handle"=w132:refnum<vi>)
            n78 = property class="DigNum (strict)"(reference=w134) -> (reference out=w136:refnum<vi>, error out=w135:errorcluster, "Value"=w133:i32)  [unwired: 1 in]
            n79 = property class="Bool (strict)"(reference=w132) -> (reference out=w130:refnum<vi>, error out=w131:errorcluster, "Value"=w129:bool)  [unwired: 1 in]
            n80 = Close Reference(reference=w136, error in (no error)=w135) -> ()  [unwired: 1 out]
            n81 = Close Reference(reference=w130, error in (no error)=w131) -> ()  [unwired: 1 out]
            n82 = case shown="True" w129 {
              tunnel: w133 -> [_ w144]
              tunnel: w138 -> [w140 w143]
              tunnel: [w140 w142] -> w137
              tunnel: [0 w141] -> w124
              frame False {
              }
              frame True {
                n83 = dll-call lib="D:/LAB-IQ 150/lib/hps_ft.dll" fn="hps_ft_deleteHandle"(error in=w143, "handle"=w144) -> (error out=w142:errorcluster, "return type"=w141:i32)  [unwired: 3 in, 1 out]
              }
            }
            n84 = Unbundle By Name(w125) -> ("Loading Com Port.deleteHandle-result"=w128:refnum<vi>)
            n85 = property class="DigNum (strict)"(reference=w128, "Value"=w124) -> (reference out=w126:refnum<vi>, error out=w127:errorcluster)  [unwired: 1 in]
            n86 = Close Reference(reference=w126, error in (no error)=w127) -> ()  [unwired: 1 out]
          }
          frame "SETZERO" {
            n87 = Unbundle By Name(w147) -> ("Loading Com Port.ft_udp_handle"=w154:refnum<vi>)
            n88 = property class="DigNum (strict)"(reference=w154) -> (reference out=w152:refnum<vi>, error out=w153:errorcluster, "Value"=w151:i32)  [unwired: 1 in]
            n89 = Close Reference(reference=w152, error in (no error)=w153) -> ()  [unwired: 1 out]
            n90 = dll-call lib="D:/LAB-IQ 150/lib/hps_ft.dll" fn="hps_ft_zero"(error in=w155, "handle"=w151) -> (error out=w145:errorcluster, "return type"=w146:i32)  [unwired: 3 in, 1 out]
            n91 = Unbundle By Name(w147) -> ("Loading Com Port.zero-return"=w150:refnum<vi>)
            n92 = property class="DigNum (strict)"(reference=w150, "Value"=w146) -> (reference out=w148:refnum<vi>, error out=w149:errorcluster)  [unwired: 1 in]
            n93 = Close Reference(reference=w148, error in (no error)=w149) -> ()  [unwired: 1 out]
          }
          frame "SETLOWPASSFILTER" {
            n94 = Unbundle By Name(w157) -> ("Loading Com Port.ft_udp_handle"=w164:refnum<vi>)
            n95 = property class="DigNum (strict)"(reference=w164) -> (reference out=w161:refnum<vi>, error out=w163:errorcluster, "Value"=w162:i32)  [unwired: 1 in]
            n96 = Close Reference(reference=w161, error in (no error)=w163) -> ()  [unwired: 1 out]
            n97 = dll-call lib="D:/LAB-IQ 150/lib/hps_ft.dll" fn="hps_ft_setLowPassFilter"(error in=w166, "handle"=w162, "level"=0) -> (error out=w165:errorcluster, "return type"=w156:i32)  [unwired: 4 in, 1 out]
            n98 = Unbundle By Name(w157) -> ("Loading Com Port.filter-return"=w160:refnum<vi>)
            n99 = property class="DigNum (strict)"(reference=w160, "Value"=w156) -> (reference out=w158:refnum<vi>, error out=w159:errorcluster)  [unwired: 1 in]
            n100 = Close Reference(reference=w158, error in (no error)=w159) -> ()  [unwired: 1 out]
          }
        }
      }
    }
    frame Error {
    }
  }
  "error IO" <- w3
